vi "ma_One-sided Cross Spectrum.vi"(8 "error in":errorcluster, 9 "dt":dbl format="%0.2f", 10 "signal Y (V)":dbl[](array[numeric]) format="%0.2f", 11 "signal X (V)":dbl[](array[numeric]) format="%0.2f") -> (0 "error out":errorcluster, 2 "df":dbl format="%0.2f", 3 "cross spectrum (V^2 rms)":cdb[](array[numeric]) format="%0.2f")   [LabVIEW 2020, in "NI_MAPro.lvlib"]
uses:
  NI_MAPro.lvlib
  NI_AALPro.lvlib
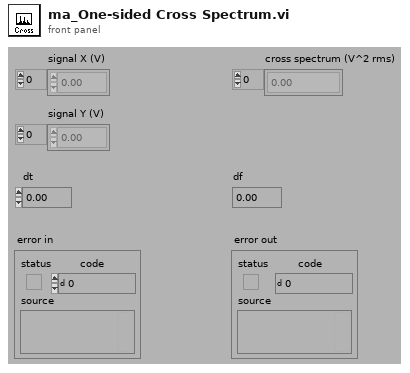
[diagram p1: front panel]
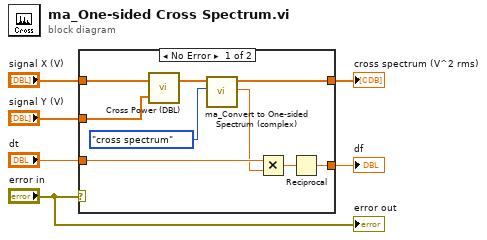
[diagram p0: block diagram]
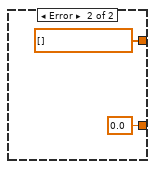
[diagram p2: hidden frame]
diagram:
  n1 = case shown="No Error" "error in" {
    tunnel: "signal X (V)" -> [w15 _]
    tunnel: "signal Y (V)" -> [w14 _]
    tunnel: "dt" -> [w13 _]
    tunnel: [w11 0.0] -> w3
    tunnel: [w9 cdb[] [] ("one-sided spectrum (complex)")] -> w2
    frame No Error {
      n2 = call "Cross Power (DBL).vi"("Y"=w14, "X"=w15) -> ("Sxy"=w10:cdb[])  [unwired: 1 out]
      n3 = call "ma_Convert to One-sided Spectrum (complex).vi"("spectrum type"=enum16{"FFT spectrum", "cross spectrum"}."cross spectrum", "two-sided spectrum (complex)"=w10) -> ("block size"=w8:dbl, "one-sided spectrum (complex)"=w9:cdb[])  [unwired: 8 out]
      n4 = Multiply(x=w13, y=w8) -> (x*y=w12:dbl)
      n5 = Reciprocal(x=w12) -> (1/x=w11:dbl)
    }
    frame Error {
    }
  }
  "cross spectrum (V^2 rms)" <- w2
  "df" <- w3
  "error out" <- "error in"
